vi "sub_SDR_mod_BPSK2QAM64.vi"(11 "Array in":i16[](array[numeric])) -> (3 "Array out":cdb[](array[numeric]))   [LabVIEW 2012]
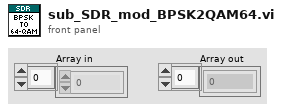
[diagram p1: front panel]
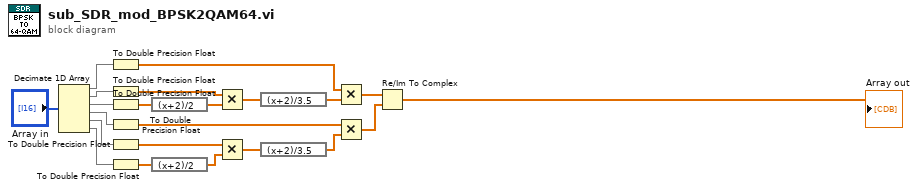
[diagram p0: block diagram]
diagram:
  n1 = Decimate 1D Array("Array in") -> (w16:i16[], w17:i16[], w18:i16[], w19:i16[], w20:i16[], w21:i16[])
  n2 = To Double Precision Float(number=w16) -> (double precision float=w8:dbl[])
  n3 = To Double Precision Float(number=w17) -> (double precision float=w9:dbl[])
  n4 = To Double Precision Float(number=w18) -> (double precision float=w11:dbl[])
  n5 = To Double Precision Float(number=w19) -> (double precision float=w2:dbl[])
  n6 = To Double Precision Float(number=w20) -> (double precision float=w3:dbl[])
  n7 = To Double Precision Float(number=w21) -> (double precision float=w5:dbl[])
  n8 = expression code="(x+2)/2"(w11) -> (w10:dbl[])
  n9 = expression code="(x+2)/2"(w5) -> (w4:dbl[])
  n10 = Multiply(x=w9, y=w10) -> (x*y=w12:dbl[])
  n11 = Multiply(x=w3, y=w4) -> (x*y=w6:dbl[])
  n12 = expression code="(x+2)/3.5"(w12) -> (w7:dbl[])
  n13 = expression code="(x+2)/3.5"(w6) -> (w1:dbl[])
  n14 = Multiply(x=w8, y=w7) -> (x*y=w13:dbl[])
  n15 = Multiply(x=w2, y=w1) -> (x*y=w14:dbl[])
  n16 = Re/Im To Complex(1:w14, 2:w13) -> (0:→"Array out":cdb[])
